vi "mnist Keras.vi"() -> ()   [LabVIEW 2018]
panel:
  in  "Python Version":enum16{"3.6", "2.7"}(ring)
  out "Status":string
  out "Predictions":sgl[](array[slide]) scale=0.0..1.0
  in  "Clear":bool
  out "Prediction":sgl
  out "Predicted Label":i32
  out "Training Results : Loss, Accuracy":dbl[](array[numeric])
  in  "Epochs":i32=3
  in  "Metrics":string="accuracy"
  in  "Loss":string="sparse_categorical_crossentropy"
  in  "Optimizer":string="adam"
  in  "stop":bool
  out "Draw pane":picture
  # "Overview: This example shows how to use the deep learning API to perform numeric classification using the Python Keras library. The model is of sequential type and is compiled using the optimizer provided by Keras. Trained using the mnist dataset, this model recognizes and classifies numbers you draw on the front panel.\nRequirements: Python 3.6 (64-bits)\nInstructions:\n1. Make sure you have TensorFlow and Keras installed in your Python environment.\n2. Open mnist Keras.vi.\n3. Run the VI. After the model has been compiled and trained, the Status indicator changes to \"Model_Predicting\".\n4. Drag the mouse into the draw pane to draw a number and the model will output the prediction."
  # "0\n1\n2\n3\n4\n5\n6\n7\n8\n9"
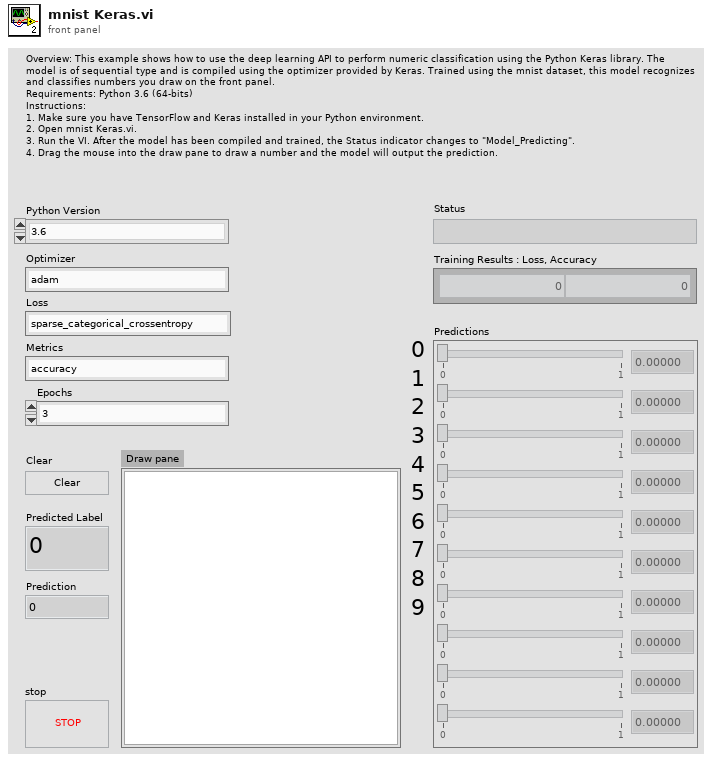
[diagram p1: front panel]
types:
  T1 = cluster{"Width":u16, "Style":enum32{"Solid", "Dash", "Dot", "DashDot", "DashDotDot"}}
  T2 = typedef "LVMouseTypeDef.ctl" = cluster{"Mouse Position":cluster{"X":i32, "Y":i32}, "Mouse Modifiers":cluster{"Button Down":bool, "Shift Mod":bool, "Menu Mod":bool, "Option Mod":bool}}
  T3 = cluster{"Button Down":bool, "Shift Mod":bool, "Menu Mod":bool, "Option Mod":bool}
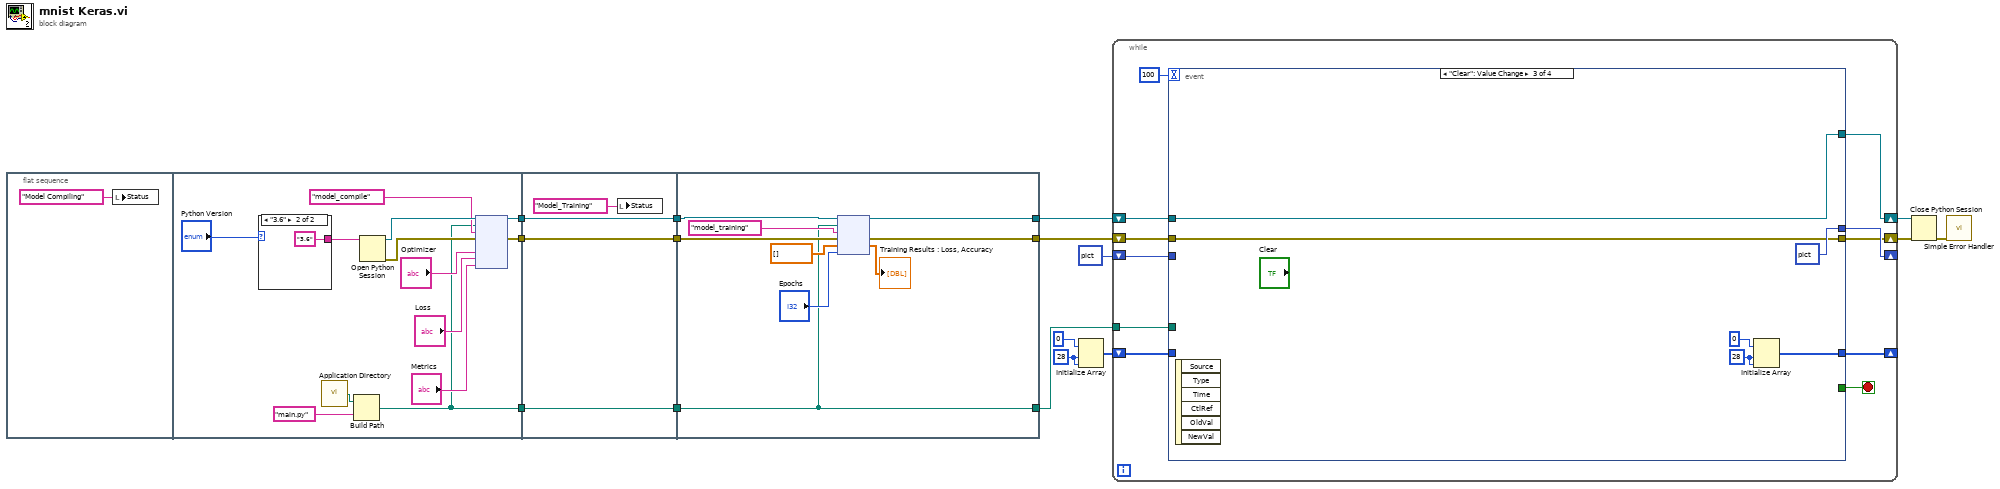
[diagram p0: block diagram]
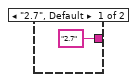
[diagram p2: hidden frame]
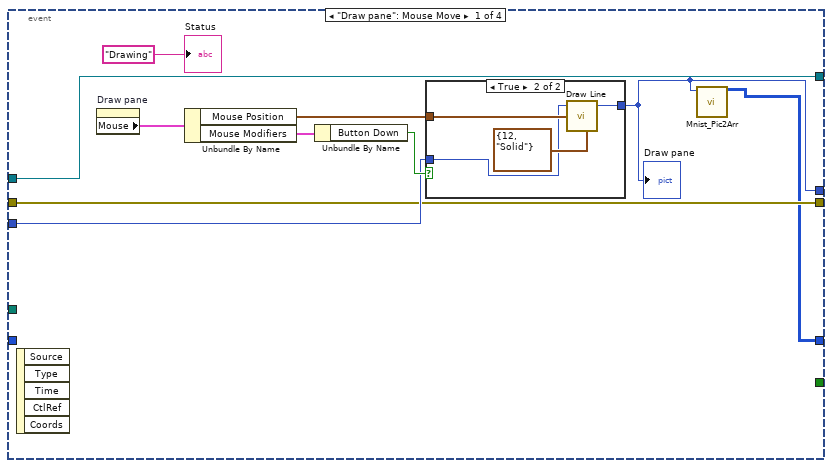
[diagram p3: hidden frame]
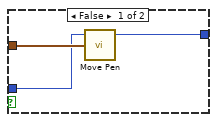
[diagram p4: hidden frame]
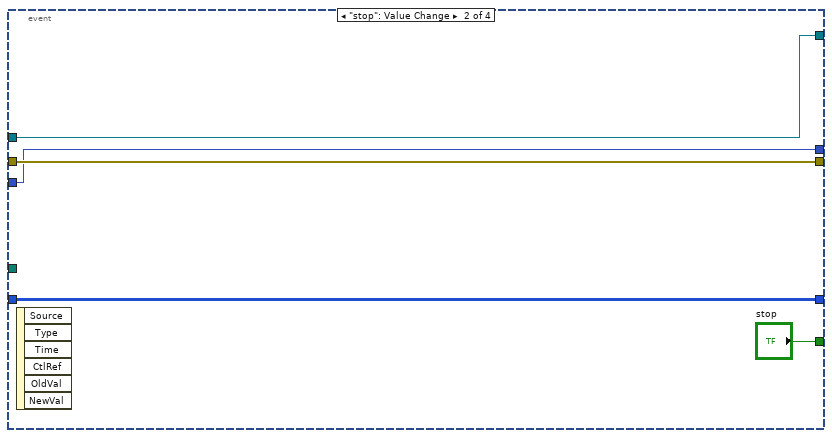
[diagram p5: hidden frame]
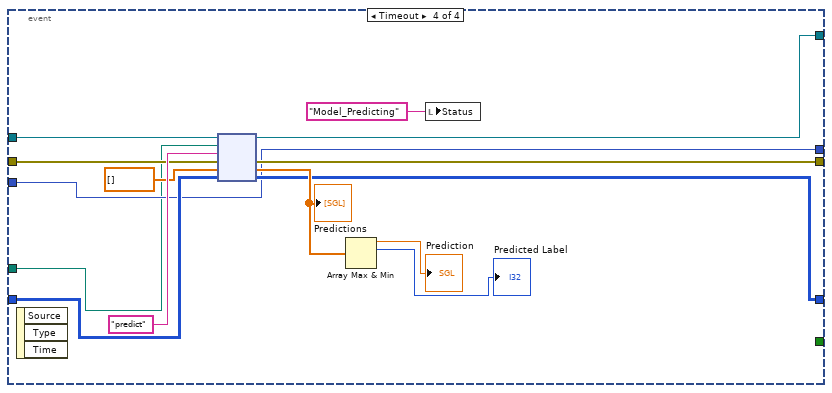
[diagram p6: hidden frame]
diagram:
  w12 = 28 ("dimension size")
  n1 = flat-sequence {
    tunnel: [w24] -> w7
    tunnel: [w23] -> w5
    tunnel: [w21] -> w3
    tunnel: w7 -> [w36]
    tunnel: [w36] -> w6
    tunnel: w5 -> [w35]
    tunnel: [w35] -> w4
    tunnel: w3 -> [w34]
    tunnel: [w34] -> w2
    tunnel: [w39] -> w9
    tunnel: w6 -> [w41]
    tunnel: w4 -> [w43]
    tunnel: w2 -> [w37]
    tunnel: [w38] -> w10
    tunnel: [w37] -> w8
    frame #0 {
      n2 = local write "Status"("Model Compiling" ("Status")) -> ()
    }
    frame #1 {
      n3 = case shown="\"3.6\"" "Python Version" {
        tunnel: ["2.7" ("python version") "3.6" ("python version")] -> w18
        frame "2.7", Default {
        }
        frame "3.6" {
        }
      }
      n4 = call <vilib>:"Application Directory.vi"() -> ("Application Directory"=w20:path)
      n5 = Build Path(base path=w20, name or relative path="main.py") -> (appended path=w21:path)
      n6 = Open Python Session(python version=w18) -> (session out=w30:refnum<k35>, error out=w29:errorcluster)  [unwired: 2 in]
      n7 = node(w30, w21, "model_compile" ("함수 이름"), w29, "Optimizer", "Loss", "Metrics") -> (w23:refnum<k35>, w24:errorcluster)  [unwired: 5 in, 2 out]
    }
    frame #2 {
      n8 = local write "Status"("Model_Training" ("Status")) -> ()
    }
    frame #3 {
      n9 = node(w43, w37, "model_training" ("함수 이름"), w41, dbl[] [], "Epochs") -> (w39:refnum<k35>, w38:errorcluster, →"Training Results : Loss, Accuracy":dbl[])  [unwired: 1 in, 2 out]
    }
  }
  n10 = Initialize Array(i64 0 ("element"), w12, w12) -> (w11:i64[][])
  n11 = while {
    shift-right: [w56] -> _
    shift-left: picture data[5B] ("empty picture") -> [w55]
    shift-right: [w48] -> _
    shift-left: w11 -> [w47]
    shift-right: [w52] -> w15
    shift-left: w9 -> [w50]
    shift-right: [w51] -> w14
    shift-left: w10 -> [w49]
    tunnel: w8 -> [w46]
    stop <- w54 stop-if-true
    n12 = event shown="[2] \"Clear\": Value Change" {
      selector: _ -> [_ _ _ _]
      dyn-events: _ -> [_ _ _ _]
      timeout: 100 -> [_ _ _ _]
      tunnel: [w57 w75 picture data[5B] ("empty picture") w87] -> w56
      tunnel: w55 -> [w62 w75 _ w87]
      tunnel: [_ "stop" _ _] -> w54
      tunnel: [w61 w77 w84 w93] -> w52
      tunnel: [w60 w76 w82 w92] -> w51
      tunnel: w50 -> [w61 w77 w84 w91]
      tunnel: w49 -> [w60 w76 w82 w90]
      tunnel: [w58 w74 w80 w88] -> w48
      tunnel: w47 -> [_ w74 _ w89]
      tunnel: w46 -> [_ _ _ w85]
      event "Draw pane": Mouse Move {
        n13 = event-data() -> ()  [unwired: 1 in, 5 out]
        n14 = property on="Draw pane" class="Pict"() -> ("Mouse"=w66:T2)  [unwired: 2 in, 2 out]
        n15 = Unbundle By Name(w66) -> ("Mouse Position"=w64:cluster{"X":i32, "Y":i32}, "Mouse Modifiers"=w65:T3)
        n16 = Unbundle By Name(w65) -> ("Button Down"=w63:bool)
        n17 = case shown="True" w63 {
          tunnel: w64 -> [w68 w73]
          tunnel: [w69 w72] -> w57
          tunnel: w62 -> [w67 w70]
          frame False {
            n18 = call <vilib>:"Move Pen.vi"("new position"=w68, "picture"=w67) -> ("new picture"=w69:picture)  [unwired: 3 in]
          }
          frame True {
            n19 = call <vilib>:"Draw Line.vi"("picture"=w70, "end point"=w73, "pen"=T1 {"Width"=12, "Style"=enum."Solid"}) -> ("new picture"=w72:picture)  [unwired: 6 in]
          }
        }
        "Draw pane" <- w57
        n20 = call "Mnist_Pic2Arr.vi"("empty picture"=w57) -> ("Img 8 bit"=w58:i64[][])  [unwired: 10 in]
        "Status" <- "Drawing" ("Status")
      }
      event "stop": Value Change {
        n21 = event-data() -> ()  [unwired: 1 in, 6 out]
      }
      event "Clear": Value Change {
        w79 = 28 ("dimension size")
        n22 = event-data() -> ()  [unwired: 1 in, 6 out]
        n23 = Initialize Array(i64 0 ("element"), w79, w79) -> (w80:i64[][])
      }
      event Timeout {
        n24 = event-data() -> ()  [unwired: 1 in, 3 out]
        n25 = node(w91, w85, "predict" ("함수 이름"), w90, sgl[] [], w89) -> (w93:refnum<k35>, w92:errorcluster, w96:sgl[], w88:i64[][])  [unwired: 2 out]
        "Predictions" <- w96
        n26 = Array Max & Min(array=w96) -> (max value=→"Prediction":sgl, max index (indices)=→"Predicted Label":i32)  [unwired: 2 out]
        n27 = local write "Status"("Model_Predicting" ("Status")) -> ()
      }
    }
  }
  n28 = Close Python Session(session in=w15, error in=w14) -> (11:w1:errorcluster)
  n29 = call <vilib>:"Simple Error Handler.vi"("error in (no error)"=w1) -> ()  [unwired: 4 in, 5 out]
